vi "LSX Get Snapshot Pos Array.vi"(0 "lLSID":i32, 1 "pdZ":dbl, 5 "lIndex":i32, 7 "pdX":dbl, 9 "pdY":dbl, 11 "error in (no error)":errorcluster, 12 "pdR":dbl) -> (3 "pdZ out":dbl, 4 "function return":i32, 8 "pdX out":dbl, 10 "pdY out":dbl, 14 "pdR out":dbl, 15 "error out":errorcluster)   [LabVIEW 2018, in "Tango.lvlib"]
doc: "TANGOAPI int TANGOCALL LSX_GetSnapshotPosArray (int lLSID, int lIndex, double *pdX, double *pdY, double *pdZ, double *pdR);"
uses:
  Tango.lvlib
  SubVIs/Tango_DLL.dll
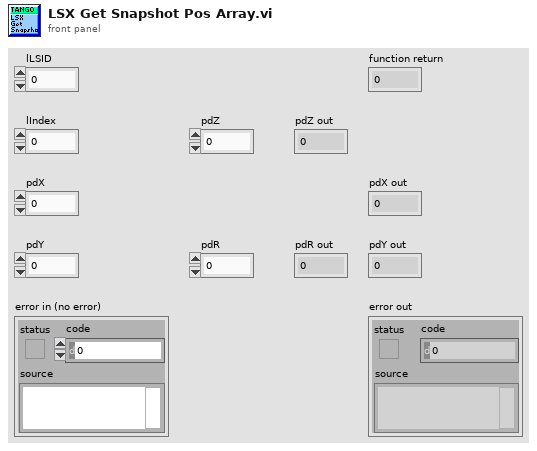
[diagram p1: front panel]
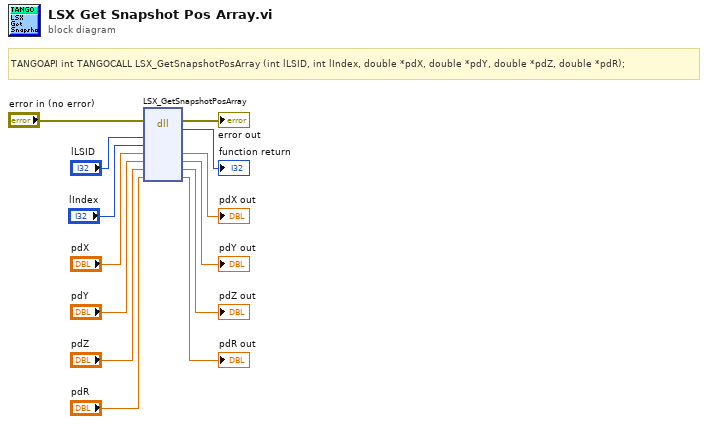
[diagram p0: block diagram]
diagram:
  # "TANGOAPI int TANGOCALL LSX_GetSnapshotPosArray (int lLSID, int lIndex, double *pdX, double *pdY, double *pdZ, double *pdR);"
  n1 = dll-call lib="C:/Users/Familie/Documents/LabviewIX81/lib/TANGO Stage/SubVIs/Tango_DLL.*" fn="LSX_GetSnapshotPosArray"(error in="error in (no error)", "lLSID"="lLSID", "lIndex"="lIndex", "pdX"="pdX", "pdY"="pdY", "pdZ"="pdZ", "pdR"="pdR") -> (error out=→"error out":errorcluster, →"function return":i32, "pdX"=→"pdX out":dbl, "pdY"=→"pdY out":dbl, "pdZ"=→"pdZ out":dbl, "pdR"=→"pdR out":dbl)  [unwired: 4 in, 1 out]
